vi "Tile naming.vi"(7 "?":T1=enum."Increment", 8 "Error In":errorcluster, 10 "Tile Num":i32) -> (0 "Error Out":errorcluster, 2 "tile":i32, 3 "slice":i32)   [LabVIEW 2018]
uses:
  Tile naming actions.ctl
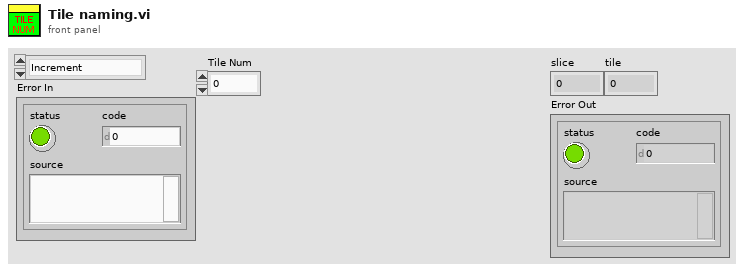
[diagram p1: front panel]
types:
  T1 = typedef "Tile naming actions.ctl" = enum16{"Export", "Increment", "Total tile num", "Init"}
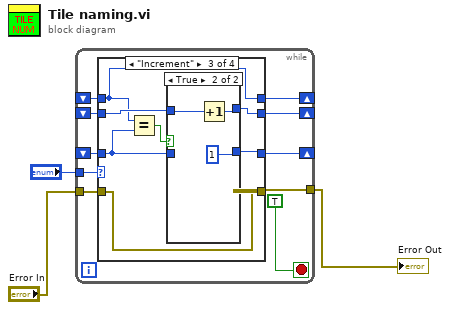
[diagram p0: block diagram]
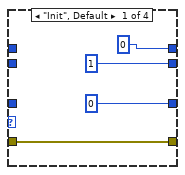
[diagram p2: hidden frame]
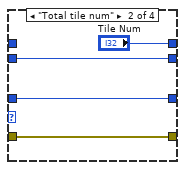
[diagram p3: hidden frame]
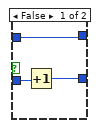
[diagram p4: hidden frame]
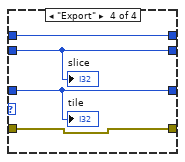
[diagram p5: hidden frame]
diagram:
  n1 = while {
    tunnel: "?" -> [w13]
    shift-right: [w11] -> _
    shift-left: _ -> [w9]
    shift-right: [w12] -> _
    shift-left: _ -> [w8]
    tunnel: "Error In" -> [w7]
    tunnel: [w6] -> w1
    shift-right: [w5] -> _
    shift-left: _ -> [w4]
    stop <- TRUE stop-if-true
    n2 = case shown="\"Increment\"" w13 {
      tunnel: [0 w18 w24 w37] -> w12
      tunnel: [1 w21 w26 w38] -> w11
      tunnel: w9 -> [_ w21 w27 w38]
      tunnel: w8 -> [_ w18 w25 w37]
      tunnel: w7 -> [w15 w20 w22 w36]
      tunnel: [w15 w20 w22 w36] -> w6
      tunnel: [0 "Tile Num" w23 w35] -> w5
      tunnel: w4 -> [_ _ w23 w35]
      frame "Init", Default {
      }
      frame "Total tile num" {
      }
      frame "Increment" {
        n3 = Equal?(x=w23, y=w25) -> (x = y?=w28:bool)
        n4 = case shown="True" w28 {
          tunnel: [w31 w33] -> w26
          tunnel: w27 -> [w31 w32]
          tunnel: w25 -> [w30 _]
          tunnel: [w29 1] -> w24
          frame False {
            n5 = Increment(x=w30) -> (x+1=w29:i32)
          }
          frame True {
            n6 = Increment(x=w32) -> (x+1=w33:i32)
          }
        }
      }
      frame "Export" {
        "slice" <- w38
        "tile" <- w37
      }
    }
  }
  "Error Out" <- w1
